vi "subGenerateDGMLNodeString.vi"(6 "Container empty?":bool, 7 "Expand?":bool, 9 "Code schema":string, 10 "Label":string, 11 "Id":string) -> (3 "Node string":string)   [LabVIEW 2020, in "DefaultExtensions.lvlib" / "CGrapherDGML.lvclass"]
uses:
  CGrapherDGML.lvclass
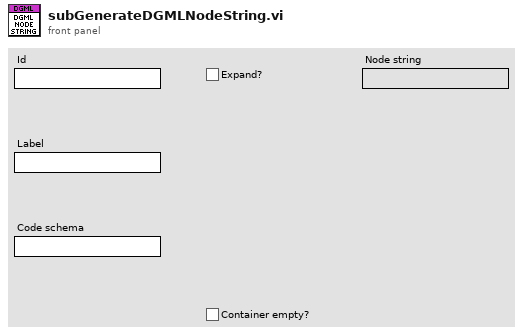
[diagram p1: front panel]
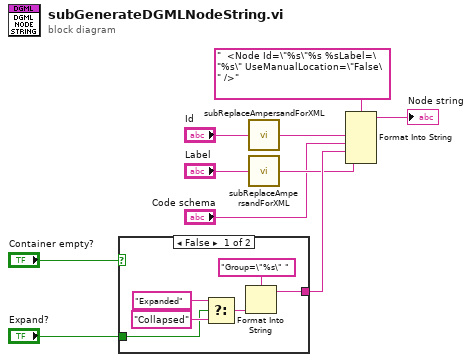
[diagram p0: block diagram]
diagram:
  n1 = case shown="False" "Container empty?" {
    tunnel: [w15 _] -> w9
    tunnel: "Expand?" -> [w13 _]
    frame False {
      n2 = Select(t="Expanded", s=w13, f="Collapsed") -> (s? t:f=w11:string)
      n3 = Format Into String(format string="Group=\"%s\" ", w11) -> (resulting string=w15:string)  [unwired: 2 in, 1 out]
    }
    frame True {
    }
  }
  n4 = call "subReplaceAmpersandForXML.vi"("String"="Id") -> ("result string"=w7:string)
  n5 = call "subReplaceAmpersandForXML.vi"("String"="Label") -> ("result string"=w8:string)
  n6 = Format Into String(format string="  <Node Id=\"%s\"%s %sLabel=\"%s\" UseManualLocation=\"False\" />", w7, "Code schema", w9, w8) -> (resulting string=→"Node string":string)  [unwired: 2 in, 1 out]
